vi "Convert Controls to Cluster.vi"(9 "Indicator Array":string[][](array[string]), 11 "Control Array":string[][](array[string])) -> (2 "Ctl Properties":T1[](array[typedef]))   [LabVIEW 2023, in "VI Properties Editor.lvlib"]
uses:
  VI Properties Editor.lvlib
  Control Properties.ctl
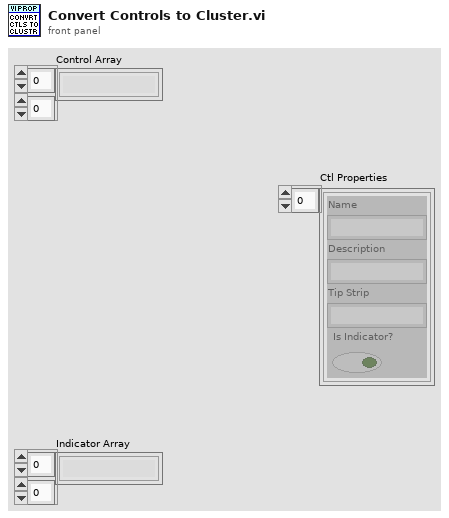
[diagram p1: front panel]
types:
  T1 = typedef "VI Properties Editor.lvlib/Control Properties.ctl" = cluster{"Name":string, "Description":string, "Tip Strip":string, "Is Indicator?":bool}
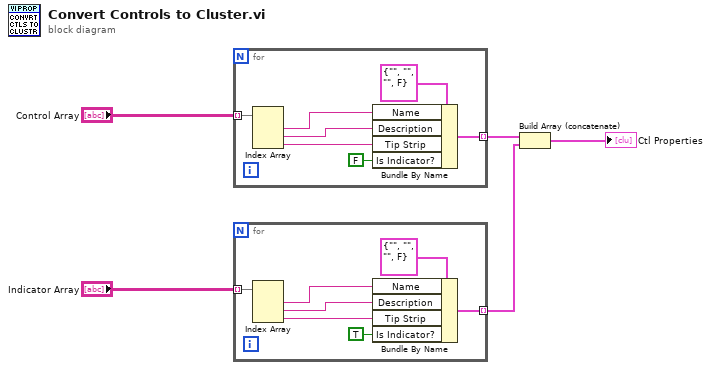
[diagram p0: block diagram]
diagram:
  n1 = for {
    tunnel: "Control Array" -> [w11] mode=indexing
    tunnel: [w6] -> w3 mode=indexing
    n2 = Index Array(array=w11) -> (element #1=w10:string, element #2=w9:string, element #3=w8:string)  [unwired: 3 in]
    n3 = Bundle By Name(cluster=T1 {"Name"="", "Description"="", "Tip Strip"="", "Is Indicator?"=FALSE} ("input cluster"), "Name"=w10, "Description"=w9, "Tip Strip"=w8, "Is Indicator?"=FALSE) -> (w6:T1)
  }
  n4 = for {
    tunnel: "Indicator Array" -> [w18] mode=indexing
    tunnel: [w13] -> w2 mode=indexing
    n5 = Index Array(array=w18) -> (element #1=w17:string, element #2=w16:string, element #3=w15:string)  [unwired: 3 in]
    n6 = Bundle By Name(cluster=T1 {"Name"="", "Description"="", "Tip Strip"="", "Is Indicator?"=FALSE} ("input cluster"), "Name"=w17, "Description"=w16, "Tip Strip"=w15, "Is Indicator?"=TRUE) -> (w13:T1)
  }
  n7 = Build Array (concatenate)(w3, w2) -> (→"Ctl Properties":T1[])
